vi "ConnectCamera.vi"() -> ()   [LabVIEW 2015]
uses:
  <vilib>/userdefined/High Color/IMAQdx.ctl
  <vilib>/MakerHub/LINX/Public/Peripherals/Digital/Digital Write 1 Chan.vi
  <vilib>/MakerHub/LINX/Public/Peripherals/Digital/Digital Read 1 Chan.vi
  <vilib>/MakerHub/LINX/Public/Peripherals/Digital/Digital Write N Chans.vi
  <vilib>/MakerHub/LINX/Public/Peripherals/Digital/Digital Read N Chans.vi
  <vilib>/MakerHub/LINX/Private/Local IO/LinxDigitalWrite.vi
  <vilib>/MakerHub/LINX/Public/Utilities/Check Channel.vi
  <vilib>/MakerHub/LINX/Private/Local IO/LinxDigitalRead.vi
  <vilib>/MakerHub/LINX/Public/Utilities/Open Serial.vi
  <vilib>/MakerHub/LINX/Private/Utilties/Generate Error.vi
  <vilib>/vision/driver/NI_Vision_Acquisition_Software.lvlib
  <vilib>/MakerHub/LINX/LMH-LINX.lvlib
  <vilib>/vision/NI_Vision_Development_Module.lvlib
panel:
  out "Arduino Error Out":errorcluster
  out "Image Masked":T1(plugin-control)
  out "JIG ARRIVE":bool
  out "Image Original":T1(plugin-control)
  in  "stop":bool
  # "Workpiece Bottom Center"
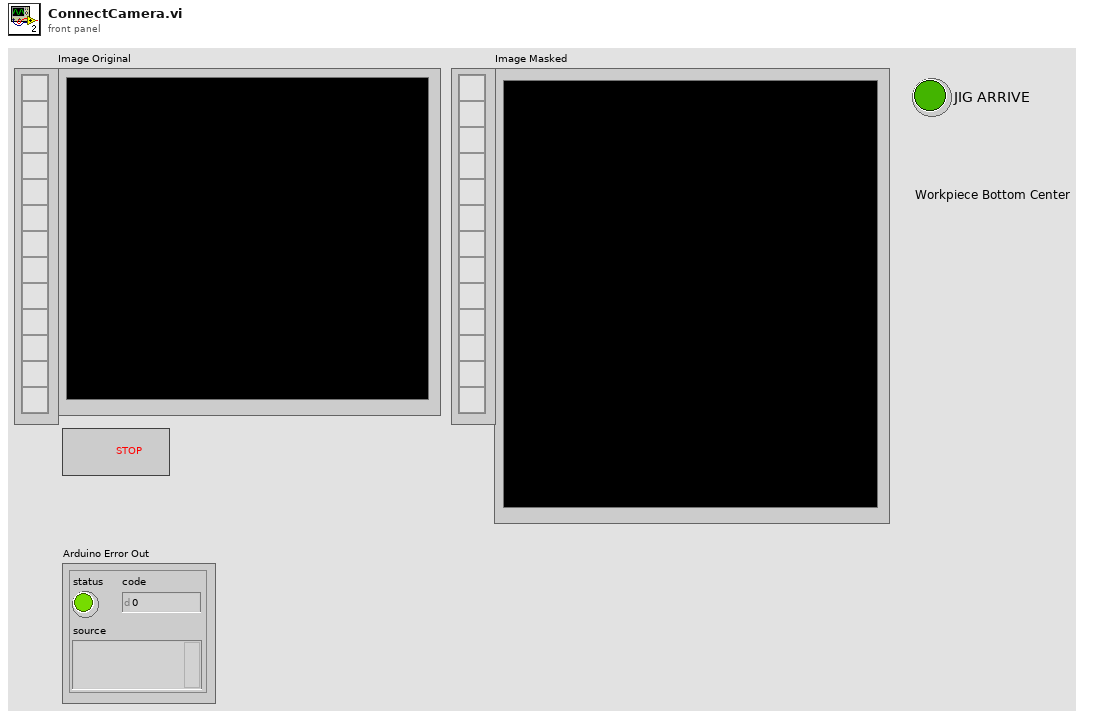
[diagram p1: front panel]
types:
  T1 = typedef "IMAQ Image.ctl" = refnum<image>
  T2 = typedef "Image Type" = u32
  T3 = typedef "IMAQdx.ctl" = refnum<k21>
  T4 = typedef "LMH-LINX.lvlib/LINX Ref.ctl" = cluster{"IO":T5, "Interface":T6, "LINX Device Config":T7}
  T5 = typedef "LMH-LINX.lvlib/Platform.ctl" = enum16{"Remote", "Local"}
  T6 = typedef "LMH-LINX.lvlib/Interface.ctl" = enum16{"Serial", "TCP"}
  T7 = typedef "LMH-LINX.lvlib/Device.lvlib/LINX Device Config.ctl" = cluster{"Interface":T6, "COM Port":refnum<visa-resource-name>, "TCP Configuration":T8, "Device Family":u8, "Device ID":u8, "Device Name":string, "TCP Ref":refnum<k5>, "Channels":T9}
  T8 = typedef "LMH-LINX.lvlib/Device.lvlib/TCP Config.ctl" = cluster{"IP Address":string, "Port":u16}
  T9 = typedef "LMH-LINX.lvlib/Channels.ctl" = cluster{"DI":u8[], "DO":u8[], "AI":u8[], "AO":u8[], "PWM":u8[], "QE":u8[], "UART":u8[], "I2C 2":u8[], "SPI":u8[], "CAN":u8[], "Servo":u8[], "AI Ref (V)":dbl, "AI Resolution (Bits)":u8, "AO Ref (V)":dbl, "AO Resolution (Bits)":u8}
  T10 = cluster{"Position":cluster{"X":sgl, "Y":sgl}, "Radius":dbl, "Score":dbl}[]
  T11 = cluster{"Circles[0]":cluster{"Position":cluster{"X":sgl, "Y":sgl}, "Radius":dbl, "Score":dbl}, "Circles[1]":cluster{"Position":cluster{"X":sgl, "Y":sgl}, "Radius":dbl, "Score":dbl}, "Circles[2]":cluster{"Position":cluster{"X":sgl, "Y":sgl}, "Radius":dbl, "Score":dbl}, "Circles[3]":cluster{"Position":cluster{"X":sgl, "Y":sgl}, "Radius":dbl, "Score":dbl}, "Circles[4]":cluster{"Position":cluster{"X":sgl, "Y":sgl}, "Radius":dbl, "Score":dbl}, "Circles[5]":cluster{"Position":cluster{"X":sgl, "Y":sgl}, "Radius":dbl, "Score":dbl}, "Circles[6]":cluster{"Position":cluster{"X":sgl, "Y":sgl}, "Radius":dbl, "Score":dbl}, "Circles[7]":cluster{"Position":cluster{"X":sgl, "Y":sgl}, "Radius":dbl, "Score":dbl}, "Circles[8]":cluster{"Position":cluster{"X":sgl, "Y":sgl}, "Radius":dbl, "Score":dbl}}
  T12 = typedef "ROI Descriptor" = cluster{"Global Rectangle":i32[], "Contours":cluster{"ID":enum32{"External", "Internal"}, "Type":u32, "Coordinates":i32[]}[]}
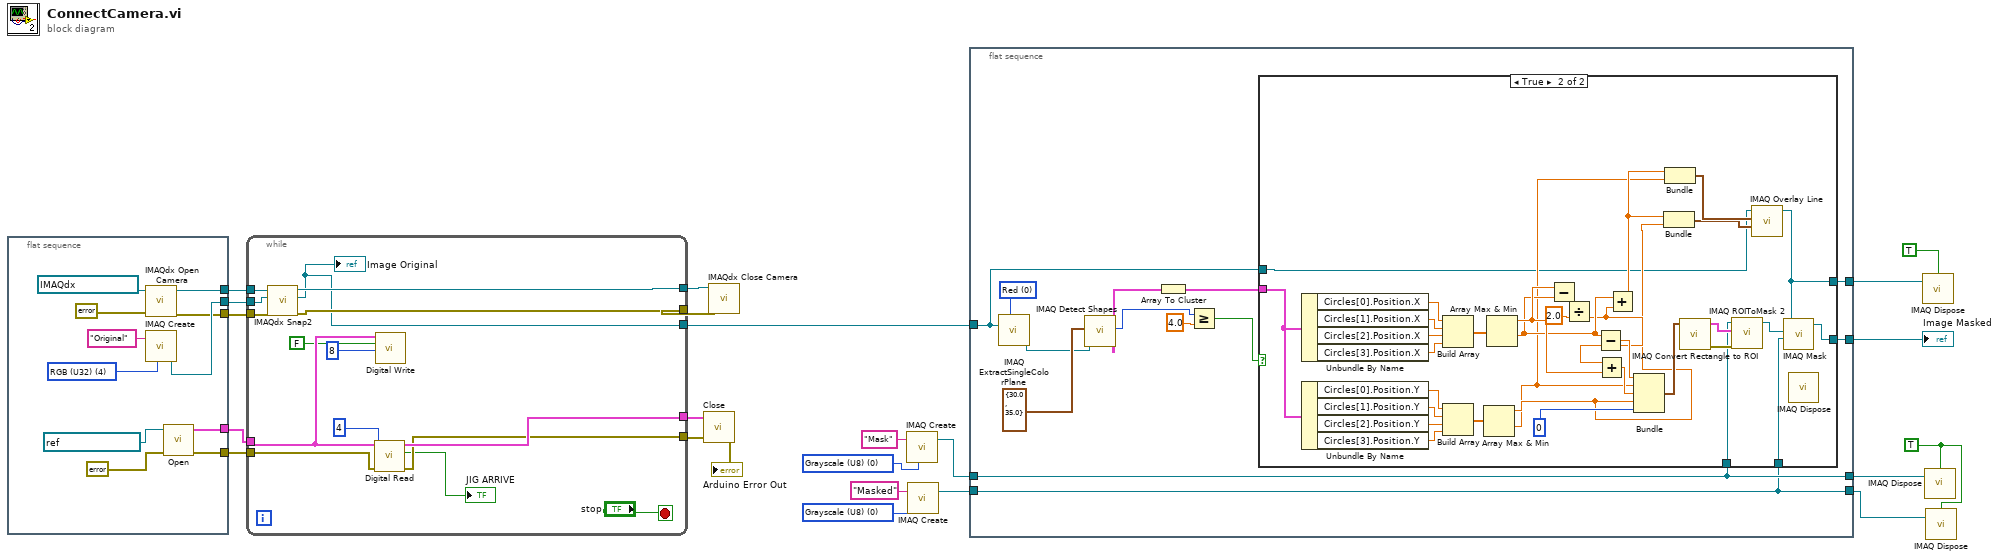
[diagram p0: block diagram]
diagram:
  w3 = TRUE ("All Images? (No)")
  w12 = T2 0 items=["Grayscale (U8)", "Grayscale (I16)", "Grayscale (SGL)", "Complex (CSG)", "RGB (U32)", "HSL (U32)", "RGB (U64)", "Grayscale (U16)"] ("Image Type")
  w14 = T2 0 items=["Grayscale (U8)", "Grayscale (I16)", "Grayscale (SGL)", "Complex (CSG)", "RGB (U32)", "HSL (U32)", "RGB (U64)", "Grayscale (U16)"] ("Image Type")
  n1 = flat-sequence {
    tunnel: [w31] -> w23
    tunnel: [w30] -> w22
    tunnel: [w29] -> w21
    tunnel: [w27] -> w18
    tunnel: [w24] -> w7
    frame #0 {
      w32 = T2 4 items=["Grayscale (U8)", "Grayscale (I16)", "Grayscale (SGL)", "Complex (CSG)", "RGB (U32)", "HSL (U32)", "RGB (U64)", "Grayscale (U16)"] ("Image Type")
      n2 = call <vilib>:"IMAQdx Open Camera.vi"("error in"=errorcluster {"status"=FALSE, "code"=0, "source"=""}, "Session In"=T3 "acA1920-25gc") -> ("error out"=w29:errorcluster, "Session Out"=w31:T3)  [unwired: 8 in]
      n3 = call "IMAQ Create"("Image Name"="Original", "Image Type"=w32) -> ("New Image"=w30:T1)  [unwired: 3 in, 1 out]
      n4 = call-poly <vilib>:"Open.vi"("Error In"=errorcluster {"status"=FALSE, "code"=0, "source"=""}, "Serial Port"=refnum<visa-resource-name> "COM4") -> ("Error Out"=w24:errorcluster, "LINX Resource"=w27:T4)  [unwired: 7 in, 1 out]
    }
  }
  n5 = while {
    tunnel: w23 -> [w49]
    tunnel: w22 -> [w48]
    tunnel: w21 -> [w47]
    tunnel: [w46] -> w20
    tunnel: [w45] -> w19
    tunnel: [w44] -> w15
    tunnel: w18 -> [w37]
    tunnel: [w42] -> w17
    tunnel: [w41] -> w16
    tunnel: w7 -> [w38]
    stop <- "stop" stop-if-true
    n6 = call <vilib>:"IMAQdx Snap2.vi"("error in"=w47, "Image In"=w48, "Session In"=w49) -> ("error out"=w45:errorcluster, "Image Out"=w44:T1, "Session Out"=w46:T3)  [unwired: 6 in]
    "Image Original" <- w44
    n7 = call-poly <vilib>:"Digital Read.vi"("Error In"=w38, "DI Channel"=u8 4, "LINX Resource"=w37) -> ("Error Out"=w41:errorcluster, "DI Value"=→"JIG ARRIVE":bool, "LINX Resource"=w42:T4)  [unwired: 6 in]
    n8 = call-poly <vilib>:"Digital Write.vi"("Output Value"=FALSE, "DO Channel"=u8 8, "LINX Resource"=w37) -> ()  [unwired: 7 in, 2 out]
  }
  n9 = call <vilib>:"Close.vi"("Error In"=w16, "LINX Resource"=w17) -> ("Error Out"=→"Arduino Error Out":errorcluster)  [unwired: 9 in]
  n10 = call <vilib>:"IMAQdx Close Camera.vi"("error in"=w19, "Session In"=w20) -> ()  [unwired: 9 in, 1 out]
  n11 = call "IMAQ Create"("Image Name"="Mask", "Image Type"=w14) -> ("New Image"=w10:T1)  [unwired: 3 in, 1 out]
  n12 = call "IMAQ Create"("Image Name"="Masked", "Image Type"=w12) -> ("New Image"=w9:T1)  [unwired: 3 in, 1 out]
  n13 = flat-sequence {
    tunnel: w15 -> [w54]
    tunnel: w10 -> [w52]
    tunnel: w9 -> [w51]
    tunnel: [w53] -> w6
    tunnel: [w52] -> w5
    tunnel: [w51] -> w4
    tunnel: [w50] -> w1
    frame #0 {
      w62 = 0 items=["Red", "Green", "Blue", "Hue", "Saturation", "Luminance", "Value", "Intensity"] ("Color Plane")
      n14 = call "IMAQ ExtractSingleColorPlane"("Color Plane"=w62, "Image Src"=w54) -> ("Image Dst Out"=w55:T1)  [unwired: 8 in, 1 out]
      n15 = call-poly "IMAQ Detect Shapes"("Circle Descriptor"=cluster{"Min Radius":dbl, "Max Radius":dbl} {"Min Radius"=30.0, "Max Radius"=35.0}, "Image"=w55) -> ("Number of Matches Returned"=w58:i32, "Circles"=w60:T10)  [unwired: 7 in, 1 out]
      n16 = Array To Cluster(array=w60) -> (cluster=w56:T11)
      n17 = Greater Or Equal?(x=w58, y=4.0) -> (x >= y?=w57:bool)
      n18 = case shown="True" w57 {
        tunnel: w56 -> [_ w84]
        tunnel: w54 -> [_ w64]
        tunnel: w52 -> [_ w80]
        tunnel: w51 -> [_ w79]
        tunnel: [_ w78] -> w53
        tunnel: [_ w63] -> w50
        frame False {
        }
        frame True {
          n19 = Unbundle By Name(w84) -> ("Circles[0].Position.X"=w85:sgl, "Circles[1].Position.X"=w86:sgl, "Circles[2].Position.X"=w87:sgl, "Circles[3].Position.X"=w88:sgl)
          n20 = Unbundle By Name(w84) -> ("Circles[0].Position.Y"=w92:sgl, "Circles[1].Position.Y"=w91:sgl, "Circles[2].Position.Y"=w90:sgl, "Circles[3].Position.Y"=w89:sgl)
          n21 = Build Array(w85, w86, w87, w88) -> (w93:sgl[])
          n22 = Build Array(w92, w91, w90, w89) -> (w94:sgl[])
          n23 = Array Max & Min(array=w94) -> (max value=w69:sgl, min value=w67:sgl)  [unwired: 2 out]
          n24 = Array Max & Min(array=w93) -> (max value=w76:sgl, min value=w71:sgl)  [unwired: 2 out]
          n25 = Subtract(x=w76, y=w71) -> (x-y=w77:sgl)
          n26 = Divide(x=w77, y=sgl 2.0) -> (x/y=w70:sgl)
          n27 = Subtract(x=w71, y=w70) -> (x-y=w72:sgl)
          n28 = Add(x=w70, y=w76) -> (x+y=w75:sgl)
          n29 = Add(x=w71, y=w70) -> (x+y=w68:sgl)
          n30 = Bundle(w72, w67, w75, w69, 0) -> (w74:cluster{sgl, sgl, sgl, sgl, i32})  [unwired: 1 in]
          n31 = Bundle(w68, w69) -> (w65:cluster{sgl, sgl})  [unwired: 1 in]
          n32 = Bundle(w68, w67) -> (w66:cluster{sgl, sgl})  [unwired: 1 in]
          n33 = call "IMAQ Convert Rectangle to ROI"("Rectangle"=w74) -> ("error out"=w83:errorcluster, "ROI Descriptor"=w82:T12)  [unwired: 8 in]
          n34 = call "IMAQ ROIToMask 2"("error in (no error)"=w83, "ROI Descriptor"=w82, "Image"=w80) -> ("Image Out"=w81:T1)  [unwired: 6 in, 2 out]
          n35 = call "IMAQ Overlay Line"("End Point"=w65, "Start Point"=w66, "Image"=w64) -> ("Image Out"=w63:T1)  [unwired: 7 in, 1 out]
          n36 = call "IMAQ Mask"("Image Dst"=w79, "Image Mask"=w81, "Image Src"=w63) -> ("Image Dst Out"=w78:T1)  [unwired: 2 in, 1 out]
        }
      }
    }
  }
  n37 = call "IMAQ Dispose"() -> ()  [unwired: 6 in, 1 out]
  n38 = call "IMAQ Dispose"("All Images? (No)"=TRUE, "Image"=w1) -> ()  [unwired: 4 in, 1 out]
  n39 = call "IMAQ Dispose"("All Images? (No)"=w3, "Image"=w5) -> ()  [unwired: 4 in, 1 out]
  n40 = call "IMAQ Dispose"("All Images? (No)"=w3, "Image"=w4) -> ()  [unwired: 4 in, 1 out]
  "Image Masked" <- w6
